vi "(auto) Set Manip.vi"(5 "G_upper bound":i32, 7 "M_lower bound":i32, 8 "error in (no error)":errorcluster) -> (0 "error out":errorcluster)   [LabVIEW 2017]
uses:
  <vilib>/myRIO/Instrument Drivers/Onboard IO/Encoder/typedefs/Encoder Reference.ctl
  <vilib>/myRIO/Common/Instrument Driver Framework/Utilities/typedefs/myRIO Generic Hardware Reference.ctl
  <vilib>/myRIO/Common/Instrument Driver Framework/Utilities/typedefs/Hardware Version Enum.ctl
  <vilib>/myRIO/Common/Instrument Driver Framework/Utilities/typedefs/myRIO v1.0 Reference.ctl
  <vilib>/myRIO/Common/Instrument Driver Framework/Utilities/typedefs/Generic FPGA Reference.ctl
  <vilib>/myRIO/Common/Instrument Driver Framework/myRIO v1.0/Encoder/typedefs/Encoder Channels Enum.ctl
  <vilib>/myRIO/Instrument Drivers/Onboard IO/PWM/typedefs/PWM Reference.ctl
  <vilib>/myRIO/Common/Instrument Driver Framework/myRIO v1.0/PWM/typedefs/PWM Channels Enum.ctl
  <vilib>/myRIO/Instrument Drivers/Onboard IO/PWM/typedefs/PWM Configuration.ctl
  <vilib>/userdefined/High Color/nirio_resource_hc.ctl
  <vilib>/myRIO/Common/Instrument Driver Framework/myRIO v1.0/Encoder/typedefs/Encoder Configuration v1.0.ctl
  <vilib>/myRIO/Common/Instrument Driver Framework/myRIO v1.0/Encoder/typedefs/Encoder Signal Mode.ctl
  <vilib>/myRIO/Instrument Drivers/Onboard IO/DIO/typedefs/DIO Reference.ctl
  <vilib>/myRIO/Common/Instrument Driver Framework/myRIO v1.0/DIO/typedefs/DIO Channels List.ctl
  <vilib>/myRIO/Common/Instrument Driver Framework/myRIO v1.0/DIO/typedefs/DIO Channels Enum.ctl
  <vilib>/myRIO/Common/Instrument Driver Framework/Utilities/vis/Is FPGA Ref Available.vi
  <vilib>/myRIO/Common/Instrument Driver Framework/myRIO v1.0/PWM/vis/myRIO v1.1 Open PWM.vi
  <vilib>/myRIO/Instrument Drivers/Onboard IO/PWM/vis/Set Duty Cycle and Frequency.vi
  <vilib>/myRIO/Common/Instrument Driver Framework/myRIO v1.0/Encoder/vis/myRIO v1.1 Open Encoder.vi
  <vilib>/myRIO/Common/Instrument Driver Framework/myRIO v1.0/DIO/vis/myRIO v1.1 Open DIO.vi
  <vilib>/myRIO/Instrument Drivers/Onboard IO/DIO/vis/Write.vi
  <vilib>/myRIO/Common/Instrument Driver Framework/Utilities/vis/Validate Channels.vi
  <vilib>/myRIO/Common/Instrument Driver Framework/myRIO v1.0/PWM/vis/myRIO v1.0 Reserve PWM.vi
  <vilib>/myRIO/Common/Instrument Driver Framework/myRIO v1.0/Encoder/vis/myRIO v1.0 Reserve Encoder.vi
  <vilib>/myRIO/Common/Instrument Driver Framework/myRIO v1.0/DIO/vis/myRIO v1.0 Reserve DIO.vi
  <vilib>/myRIO/Common/Instrument Driver Framework/myRIO v1.0/PWM/vis/myRIO v1.0 Build MUX Configuration PWM.vi
  <vilib>/myRIO/Common/Instrument Driver Framework/myRIO v1.0/Resource Manager/vis/myRIO v1.0 Reserve Channel List.vi
  <vilib>/myRIO/Common/Instrument Driver Framework/myRIO v1.0/Encoder/vis/myRIO v1.0 Build MUX Configuration Encoder.vi
  <vilib>/myRIO/Common/Instrument Driver Framework/myRIO v1.0/DIO/vis/myRIO v1.0 Build MUX Configuration DIO.vi
  <vilib>/myRIO/Common/Instrument Driver Framework/myRIO v1.0/Resource Manager/vis/myRIO v1.0 Create Configuration List.vi
  <vilib>/myRIO/Common/Instrument Driver Framework/myRIO v1.0/Resource Manager/vis/myRIO v1.0 Reserve Channel.vi
  <vilib>/myRIO/Common/Instrument Driver Framework/myRIO v1.0/Resource Manager/vis/myRIO v1.0 Unreserve Channel.vi
  <vilib>/myRIO/Common/Instrument Driver Framework/myRIO v1.0/Resource Manager/vis/myRIO v1.0 Build Mutex Name.vi
  <vilib>/Utility/VariantDataType/GetNumericInfo.vi
  <vilib>/Utility/error.llb/Error Cluster From Error Code.vi
  <vilib>/myRIO/Common/Instrument Driver Framework/myRIO v1.0/myRIO v1.1 Open.vi
  <vilib>/myRIO/Common/Instrument Driver Framework/Utilities/vis/IO Manager.vi
  <vilib>/myRIO/Common/Instrument Driver Framework/Utilities/vis/Configuration Manager.vi
  <vilib>/myRIO/Common/Instrument Driver Framework/myRIO v1.0/Resource Manager/vis/myRIO v1.0 Configure IO.vi
  <vilib>/myRIO/Common/Instrument Driver Framework/myRIO v1.0/myRIO v1.0 Close.vi
  <vilib>/myRIO/Common/Instrument Driver Framework/myRIO v1.0/Encoder/vis/myRIO v1.0 Configure Encoder.vi
  <vilib>/myRIO/Common/Instrument Driver Framework/myRIO v1.0/Encoder/vis/myRIO v1.0 Reset Encoder.vi
  <vilib>/myRIO/Common/Instrument Driver Framework/myRIO v1.0/PWM/vis/myRIO v1.0 Write PWM.vi
  <vilib>/myRIO/Common/Instrument Driver Framework/myRIO v1.0/Encoder/vis/myRIO v1.0 Read Encoder.vi
  <vilib>/myRIO/Common/Instrument Driver Framework/myRIO v1.0/DIO/vis/myRIO v1.0 Write DIO.vi
  <vilib>/myRIO/Instrument Drivers/Onboard IO/Encoder/vis/myRIO Encoder Open.xnode
  <vilib>/myRIO/Express VI/Onboard IO/PWM/PWM Express VI.xnode
  <vilib>/myRIO/Instrument Drivers/Onboard IO/PWM/vis/myRIO PWM Open.xnode
  <vilib>/myRIO/Express VI/Onboard IO/DO/DO Express VI.xnode
  <vilib>/myRIO/Instrument Drivers/Onboard IO/DIO/vis/myRIO DIO Open.xnode
  <vilib>/myRIO/Instrument Drivers/Onboard IO/Encoder/Encoder.lvlib
  <vilib>/myRIO/Instrument Drivers/Onboard IO/DIO/DIO.lvlib
  <vilib>/myRIO/Instrument Drivers/Onboard IO/PWM/PWM.lvlib
panel:
  in  "Encoder Ref In":T1
  in  "G_PWM":dbl=0.4
  in  "M_PWM":dbl=0.4
  in  "resetM?":bool
  out "G enc val":i32
  out "G+":bool
  in  "stopG":bool
  in  "G- (B/DIO7 (Pin 25))":bool
  in  "G+ (B/DIO13 (Pin 26))":bool
  out "ArrG_enc_val":i32[](array[numeric])
  out "reversedG":bool
  out "M enc val":i32
  in  "stopM":bool
  out "M+":bool
  in  "offset":i32=50
  in  "frames to pass":i32=100
  in  "iterations control":i32=10
  in  "M+ (B/DIO5 (Pin 21))":bool
  in  "M- (B/DIO6 (Pin 23))":bool
  in  "offset for Extra Stop":i32=100
  out "ArrM_enc_val":i32[](array[numeric])
  in  "def it":i32=100
  out "reversedM":bool
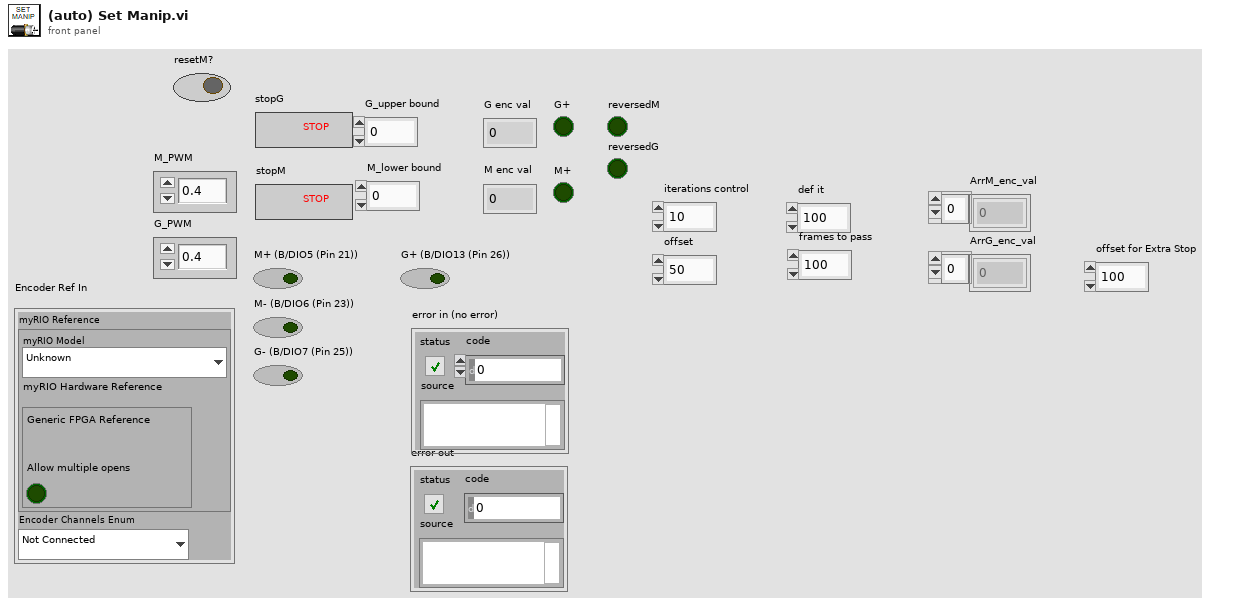
[diagram p1: front panel]
types:
  T1 = typedef "Encoder.lvlib/Encoder Reference.ctl" = cluster{"myRIO Reference":T2, "Encoder Channels Enum":T6}
  T2 = typedef "myRIO Generic Hardware Reference.ctl" = cluster{"myRIO Model":T3, "myRIO Hardware Reference":T4}
  T3 = typedef "Hardware Version Enum.ctl" = enum16{"Unknown", "myRIO-1900", "myRIO-1950", "roboRIO", "NI ELVIS RIO CM"}
  T4 = typedef "myRIO v1.0 Reference.ctl" = cluster{"Generic FPGA Reference":T5, "Allow multiple opens":bool}
  T5 = typedef "Generic FPGA Reference.ctl" = refnum<k20>
  T6 = typedef "Encoder Channels Enum.ctl" = enum16{"Not Connected", "C/ENC0", "C/ENC1", "A/ENC", "B/ENC", "DIO/ENC0", "DIO/ENC1", "DIO/ENC2", "DIO/ENC3", "DIO/ENC4"}
  T7 = typedef "PWM.lvlib/PWM Reference.ctl" = cluster{"myRIO Reference":T2, "PWM Channels Enum":T8, "PWM Configuration":T9}
  T8 = typedef "PWM Channels Enum.ctl" = enum16{"Not Connected", "C/PWM0", "C/PWM1", "A/PWM0", "A/PWM1", "A/PWM2", "B/PWM0", "B/PWM1", "B/PWM2", "PWM/PWM0", "PWM/PWM1", "PWM/PWM2", "PWM/PWM3", "PWM/PWM4", "PWM/PWM5", "PWM/PWM6", "PWM/PWM7", "PWM/PWM8", "PWM/PWM9"}
  T9 = typedef "PWM.lvlib/PWM Configuration.ctl" = cluster{"Frequency":dbl, "Duty Cycle":dbl}
  T10 = typedef "nirio_resource_hc.ctl" = tag
  T11 = typedef "DIO.lvlib/DIO Reference.ctl" = cluster{"myRIO Reference":T2, "DIO Channels List":T12}
  T12 = typedef "DIO Channels List.ctl" = T13[]
  T13 = typedef "DIO Channels Enum.ctl" = enum16{"Not Connected", "C/DIO0", "C/DIO1", "C/DIO2", "C/DIO3", "C/DIO4", "C/DIO5", "C/DIO6", "C/DIO7", "A/DIO0", "A/DIO1", "A/DIO2", "A/DIO3", "A/DIO4", "A/DIO5", "A/DIO6", "A/DIO7", "A/DIO8", "A/DIO9", "A/DIO10", "A/DIO11", "A/DIO12", "A/DIO13", "A/DIO14", "A/DIO15", "B/DIO0", "B/DIO1", "B/DIO2", "B/DIO3", "B/DIO4", "B/DIO5", "B/DIO6", "B/DIO7", "B/DIO8", "B/DIO9", "B/DIO10", "B/DIO11", "B/DIO12", "B/DIO13", "B/DIO14", "B/DIO15", "LED0", "LED1", "LED2", "LED3", "Button0", "DIO/DIO0", "DIO/DIO1", "DIO/DIO2", "DIO/DIO3", "DIO/DIO4", "DIO/DIO5", "DIO/DIO6", "DIO/DIO7", "DIO/DIO8", "DIO/DIO9", "SPI/CS0", "SPI/CS1", "SPI/CS2", "SPI/CS3", "LED RADIO (Green)", "LED RADIO (Red)", "LED COMM (Green)", "LED COMM (Red)", "LED MODE (Green)", "LED MODE (Red)"}
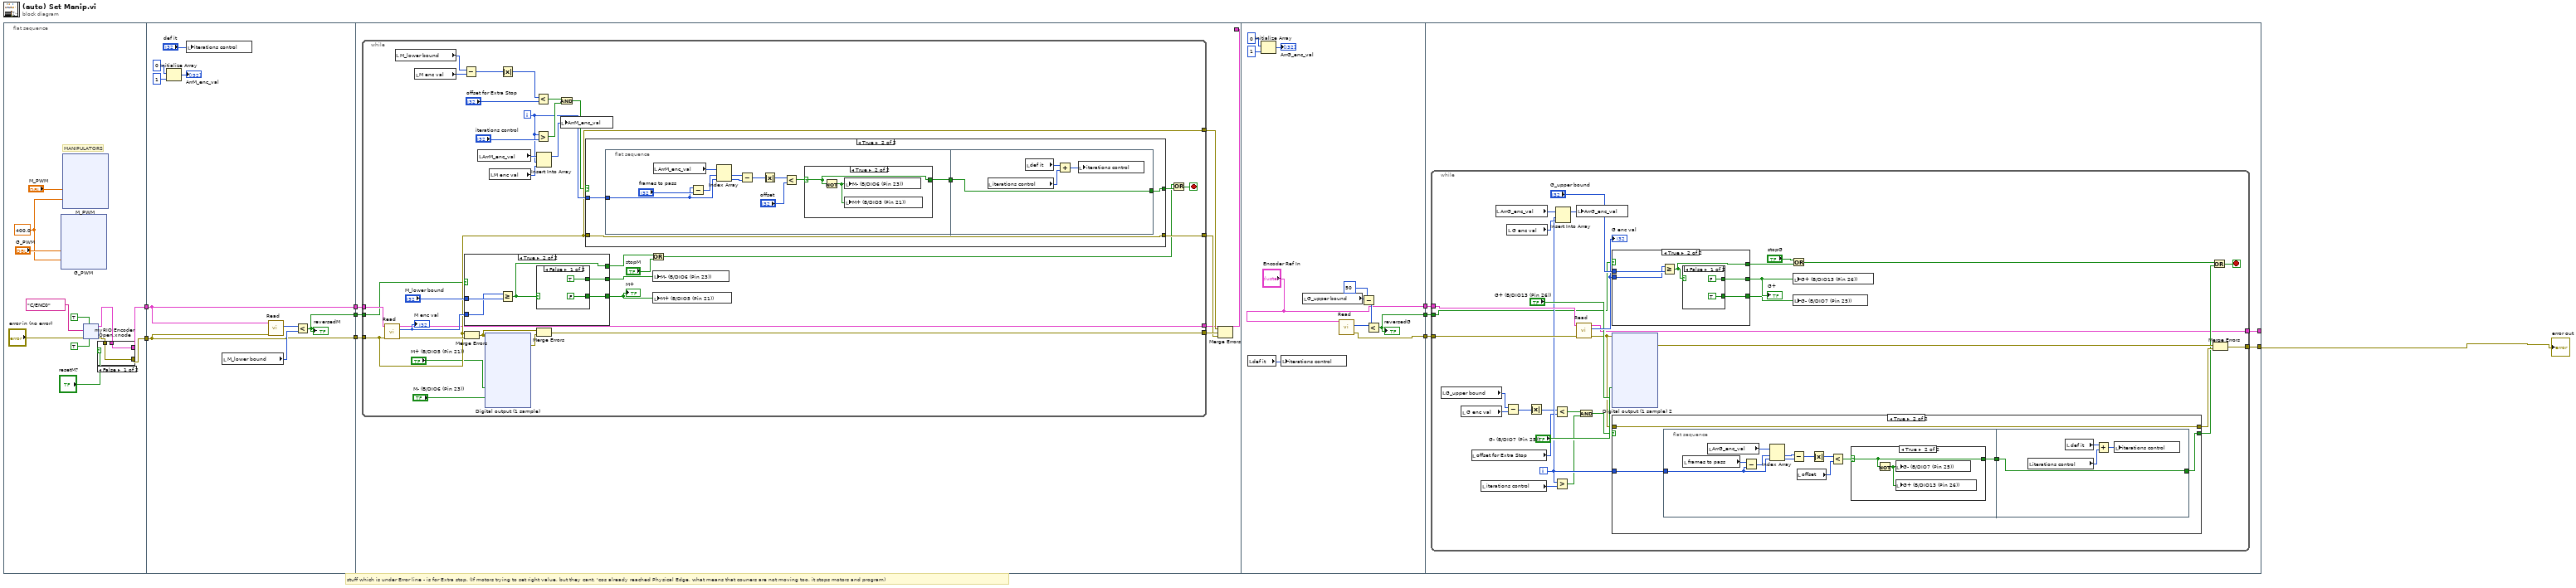
[diagram p0: block diagram]
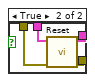
[diagram p2: hidden frame]
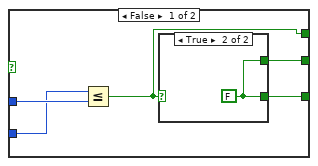
[diagram p5: hidden frame]
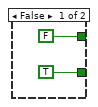
[diagram p6: hidden frame]
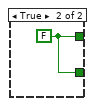
[diagram p7: hidden frame]
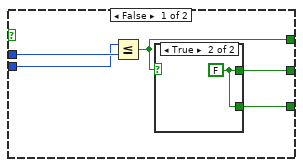
[diagram p10: hidden frame]
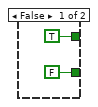
[diagram p11: hidden frame]
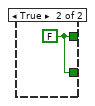
[diagram p12: hidden frame]
diagram:
  # "stuff which is under Error line - is for Extra stop. (If motors trying to set right value, but they cant, 'cos already reached Physical Edge, what means that couners are not moving too, it stops motors and program)"
  n1 = flat-sequence {
    tunnel: [w15] -> w3
    tunnel: [w14] -> w2
    tunnel: [w120] -> w9
    tunnel: [w119] -> w8
    tunnel: [w121] -> w7
    tunnel: w3 -> [w120]
    tunnel: w2 -> [w119]
    tunnel: w9 -> [w134]
    tunnel: w8 -> [w131]
    tunnel: w7 -> [w129]
    tunnel: [w128] -> _
    tunnel: [w247] -> w6
    tunnel: ["Encoder Ref In"] -> w5
    tunnel: [w248] -> w4
    tunnel: w6 -> [w259]
    tunnel: w5 -> [w258]
    tunnel: [w257] -> w1
    tunnel: w4 -> [w256]
    tunnel: [w255] -> _
    frame #0 {
      w10 = 400.0 ("Frequency [Hz]")
      # "MANIPULATORS"
      n2 = xnode "G_PWM"("Duty Cycle"="G_PWM", "Frequency [Hz]"=w10) -> ()  [unwired: 1 in, 1 out]
      n3 = xnode "M_PWM"("Duty Cycle"="M_PWM", "Frequency [Hz]"=w10) -> ()  [unwired: 1 in, 1 out]
      n4 = xnode "myRIO Encoder Open.xnode"("error in (no error)"="error in (no error)", "Allow multiple opens?"=TRUE, "Channel Name"=tag "C/ENC0", "Start Counter"=TRUE) -> ("error out"=w16:errorcluster, "Encoder Ref Out"=w17:T1)  [unwired: 1 in]
      n5 = case shown="False" "resetM?" {
        tunnel: w17 -> [w93 w97]
        tunnel: w16 -> [w92 w96]
        tunnel: [w92 w95] -> w15
        tunnel: [w93 w94] -> w14
        frame False {
        }
        frame True {
          n6 = call <vilib>:"Reset.vi"("error in (no error)"=w96, "Encoder Ref In"=w97) -> ("error out"=w95:errorcluster, "Encoder Ref Out"=w94:T1)  [unwired: 8 in]
        }
      }
    }
    frame #1 {
      n7 = Initialize Array(0 ("dimension size"), 1 ("dimension size")) -> (→"ArrM_enc_val":i32[])
      n8 = local write "iterations control"("def it") -> ()
      n9 = local read "M_lower bound"() -> (w122:i32)
      n10 = call <vilib>:"Read.vi"("error in (no error)"=w120, "Encoder Ref In"=w119) -> ("Counter Value"=w123:i32)  [unwired: 5 in, 4 out]
      n11 = Less?(x=w123, y=w122) -> (x < y?=w121:bool)
      "reversedM" <- w121
    }
    frame #2 {
      n12 = while {
        tunnel: w134 -> [w151]
        tunnel: [w151] -> w133
        tunnel: [w166] -> w132
        tunnel: w131 -> [w165]
        tunnel: [w150] -> w130
        tunnel: w129 -> [w136]
        tunnel: [w135] -> w128
        i -> [w152]
        stop <- w148 stop-if-true
        n13 = call <vilib>:"Read.vi"("error in (no error)"=w151, "Encoder Ref In"=w165) -> ("error out"=w164:errorcluster, "Counter Value"=w163:i32, "Encoder Ref Out"=w135:T1)  [unwired: 5 in, 2 out]
        "M enc val" <- w163
        n14 = local read "M_lower bound"() -> (w141:i32)
        n15 = local read "M enc val"() -> (w142:i32)
        n16 = Subtract(x=w141, y=w142) -> (x-y=w139:i32)
        n17 = case shown="True" w136 {
          tunnel: "M_lower bound" -> [w196 w204]
          tunnel: [w192 w200] -> w159
          tunnel: w163 -> [w195 w203]
          tunnel: [w194 w201] -> w145
          tunnel: [w193 w202] -> w144
          frame False {
            n18 = Less Or Equal?(x=w195, y=w196) -> (x <= y?=w192:bool)
            n19 = case shown="True" w192 {
              tunnel: [TRUE w199] -> w194
              tunnel: [FALSE w199] -> w193
              frame False {
              }
              frame True {
                w199 = FALSE
              }
            }
          }
          frame True {
            n20 = Greater Or Equal?(x=w203, y=w204) -> (x >= y?=w200:bool)
            n21 = case shown="False" w200 {
              tunnel: [TRUE ("M- (B/DIO6 (Pin 23))") w207] -> w202
              tunnel: [FALSE ("M- (B/DIO6 (Pin 23))") w207] -> w201
              frame False {
              }
              frame True {
                w207 = FALSE
              }
            }
          }
        }
        "M+" <- w145
        n22 = Merge Errors(w151, w164) -> (w160:errorcluster)
        n23 = local read "ArrM_enc_val"() -> (w155:i32[])
        n24 = xnode "Digital output (1 sample)"("M+ (B/DIO5 (Pin 21))"="M+ (B/DIO5 (Pin 21))", "M- (B/DIO6 (Pin 23))"="M- (B/DIO6 (Pin 23))", "error in (no error)"=w160) -> ("error out"=w161:errorcluster)
        n25 = local read "M enc val"() -> (w153:i32)
        n26 = Absolute Value(x=w139) -> (abs(x)=w137:i32)
        n27 = Less?(x=w137, y="offset for Extra Stop") -> (x < y?=w140:bool)
        n28 = Greater?(x=w152, y="iterations control") -> (0:w157:bool)
        n29 = Insert Into Array(array=w155, index=w152, new element=w153) -> (w154:i32[])
        n30 = Merge Errors(w160, w161) -> (w166:errorcluster)
        n31 = And(x=w140, y=w157) -> (x .and. y?=w143:bool)
        n32 = local write "ArrM_enc_val"(w154) -> ()
        n33 = case shown="True" w143 {
          selector: w143 -> [w168 _]
          tunnel: w152 -> [_ w173]
          tunnel: w151 -> [w169 w172]
          tunnel: [w169 w172] -> w150
          tunnel: [w168 w170] -> w158
          frame False {
          }
          frame True {
            n34 = flat-sequence {
              tunnel: w173 -> [w181]
              tunnel: [w174] -> w171
              tunnel: [w188] -> w170
              tunnel: w171 -> [w188]
              frame #0 {
                n35 = local read "ArrM_enc_val"() -> (w184:i32[])
                n36 = Subtract(x=w181, y="frames to pass") -> (x-y=w182:i32)
                n37 = Index Array(array=w184, index #1=w182, index #2=w181) -> (element #1=w180:i32, element #2=w179:i32)
                n38 = Subtract(x=w180, y=w179) -> (x-y=w178:i32)
                n39 = Absolute Value(x=w178) -> (abs(x)=w177:i32)
                n40 = Less?(x=w177, y="offset") -> (x < y?=w175:bool)
                n41 = case shown="True" w175 {
                  selector: w175 -> [w185 w186]
                  tunnel: [w185 w186] -> w174
                  frame False {
                  }
                  frame True {
                    n42 = Not(x=w186) -> (.not. x?=w187:bool)
                    n43 = local write "M- (B/DIO6 (Pin 23))"(w187) -> ()
                    n44 = local write "M+ (B/DIO5 (Pin 21))"(w187) -> ()
                  }
                }
              }
              frame #1 {
                n45 = local read "iterations control"() -> (w191:i32)
                n46 = local read "def it"() -> (w189:i32)
                n47 = Add(x=w189, y=w191) -> (x+y=w190:i32)
                n48 = local write "iterations control"(w190) -> ()
              }
            }
          }
        }
        n49 = Or(x=w159, y="stopM") -> (x .or. y?=w149:bool)
        n50 = local write "M- (B/DIO6 (Pin 23))"(w144) -> ()
        n51 = local write "M+ (B/DIO5 (Pin 21))"(w145) -> ()
        n52 = Or(x=w149, y=w158) -> (x .or. y?=w148:bool)
      }
      n53 = Merge Errors(w133, w132, w130) -> ()  [unwired: 1 out]
    }
    frame #3 {
      n54 = local read "def it"() -> (w252:i32)
      n55 = Initialize Array(0 ("dimension size"), 1 ("dimension size")) -> (→"ArrG_enc_val":i32[])
      n56 = local write "iterations control"(w252) -> ()
      n57 = local read "G_upper bound"() -> (w249:i32)
      n58 = call <vilib>:"Read.vi"("Encoder Ref In"="Encoder Ref In") -> ("error out"=w247:errorcluster, "Counter Value"=w250:i32)  [unwired: 6 in, 3 out]
      n59 = Subtract(x=w249, y=50) -> (x-y=w246:i32)
      n60 = Less?(x=w250, y=w246) -> (x < y?=w248:bool)
      "reversedG" <- w248
    }
    frame #4 {
      n61 = while {
        tunnel: w259 -> [w289]
        tunnel: [w274] -> w257
        tunnel: w258 -> [w285]
        tunnel: w256 -> [w261]
        tunnel: [w260] -> w255
        i -> [w276]
        stop <- w271 stop-if-true
        n62 = local read "G_upper bound"() -> (w265:i32)
        n63 = local read "G enc val"() -> (w266:i32)
        n64 = local read "offset for Extra Stop"() -> (w264:i32)
        n65 = local read "iterations control"() -> (w278:i32)
        n66 = local read "ArrG_enc_val"() -> (w279:i32[])
        n67 = Subtract(x=w265, y=w266) -> (x-y=w267:i32)
        n68 = local read "G enc val"() -> (w280:i32)
        n69 = Absolute Value(x=w267) -> (abs(x)=w262:i32)
        n70 = Less?(x=w262, y=w264) -> (x < y?=w263:bool)
        n71 = Greater?(x=w276, y=w278) -> (0:w272:bool)
        n72 = Insert Into Array(array=w279, index=w276, new element=w280) -> (w277:i32[])
        n73 = local write "ArrG_enc_val"(w277) -> ()
        n74 = call <vilib>:"Read.vi"("error in (no error)"=w289, "Encoder Ref In"=w285) -> ("error out"=w275:errorcluster, "Counter Value"=w290:i32, "Encoder Ref Out"=w260:T1)  [unwired: 5 in, 2 out]
        "G enc val" <- w290
        n75 = And(x=w263, y=w272) -> (x .and. y?=w268:bool)
        n76 = case shown="True" w261 {
          tunnel: "G_upper bound" -> [w320 w328]
          tunnel: w290 -> [w319 w327]
          tunnel: [w316 w324] -> w287
          tunnel: [w318 w325] -> w282
          tunnel: [w317 w326] -> w281
          frame False {
            n77 = Less Or Equal?(x=w319, y=w320) -> (x <= y?=w316:bool)
            n78 = case shown="True" w316 {
              tunnel: [TRUE w323] -> w318
              tunnel: [FALSE w323] -> w317
              frame False {
              }
              frame True {
                w323 = FALSE
              }
            }
          }
          frame True {
            n79 = Greater Or Equal?(x=w327, y=w328) -> (x >= y?=w324:bool)
            n80 = case shown="False" w324 {
              tunnel: [TRUE w331] -> w326
              tunnel: [FALSE w331] -> w325
              frame False {
              }
              frame True {
                w331 = FALSE
              }
            }
          }
        }
        "G+" <- w282
        n81 = xnode "Digital output (1 sample) 2"("G- (B/DIO7 (Pin 25))"="G- (B/DIO7 (Pin 25))", "G+ (B/DIO13 (Pin 26))"="G+ (B/DIO13 (Pin 26))", "error in (no error)"=w275) -> ("error out"=w286:errorcluster)
        n82 = case shown="True" w268 {
          selector: w268 -> [w292 _]
          tunnel: w276 -> [_ w297]
          tunnel: w275 -> [w293 w296]
          tunnel: [w293 w296] -> w273
          tunnel: [w292 w295] -> w269
          frame False {
          }
          frame True {
            n83 = flat-sequence {
              tunnel: w297 -> [w303]
              tunnel: [w298] -> w294
              tunnel: [w312] -> w295
              tunnel: w294 -> [w312]
              frame #0 {
                n84 = local read "frames to pass"() -> (w301:i32)
                n85 = local read "ArrG_enc_val"() -> (w308:i32[])
                n86 = Subtract(x=w301, y=w303) -> (x-y=w302:i32)
                n87 = Index Array(array=w308, index #1=w302, index #2=w303) -> (element #1=w305:i32, element #2=w300:i32)
                n88 = Subtract(x=w305, y=w300) -> (x-y=w307:i32)
                n89 = local read "offset"() -> (w299:i32)
                n90 = Absolute Value(x=w307) -> (abs(x)=w306:i32)
                n91 = Less?(x=w306, y=w299) -> (x < y?=w304:bool)
                n92 = case shown="True" w304 {
                  selector: w304 -> [w309 w310]
                  tunnel: [w309 w310] -> w298
                  frame False {
                  }
                  frame True {
                    n93 = Not(x=w310) -> (.not. x?=w311:bool)
                    n94 = local write "G- (B/DIO7 (Pin 25))"(w311) -> ()
                    n95 = local write "G+ (B/DIO13 (Pin 26))"(w311) -> ()
                  }
                }
              }
              frame #1 {
                n96 = local read "iterations control"() -> (w314:i32)
                n97 = local read "def it"() -> (w313:i32)
                n98 = Add(x=w313, y=w314) -> (x+y=w315:i32)
                n99 = local write "iterations control"(w315) -> ()
              }
            }
          }
        }
        n100 = Or(x="stopG", y=w287) -> (x .or. y?=w270:bool)
        n101 = local write "G+ (B/DIO13 (Pin 26))"(w282) -> ()
        n102 = local write "G- (B/DIO7 (Pin 25))"(w281) -> ()
        n103 = Or(x=w270, y=w269) -> (x .or. y?=w271:bool)
        n104 = Merge Errors(w286, w273) -> (w274:errorcluster)
      }
    }
  }
  "error out" <- w1
